vi "Get All Motors.vi"(8 "error in (no error)":errorcluster, 11 "MotionSystem in":refnum<class "MotionSystem.lvclass">) -> (0 "error out":errorcluster, 1 "motors":refnum<class "Motor.lvclass">[](array[class]), 2 "labels":string[](array[string]), 3 "MotionSystem out":refnum<class "MotionSystem.lvclass">)   [LabVIEW 2016, in "MotionSystem.lvlib" / "MotionSystem.lvclass"]
uses:
  <userlib>/Common Components/Hardware/Abstract System/MotionSystem/MotionSystem/MotionSystem.lvclass
  <userlib>/Common Components/Hardware/Motor/Motor/Motor.lvclass
  <userlib>/Common Components/Hardware/Abstract System/MotionSystem/MotionSystem/MotionSystem.lvclass/MotionSystem.ctl
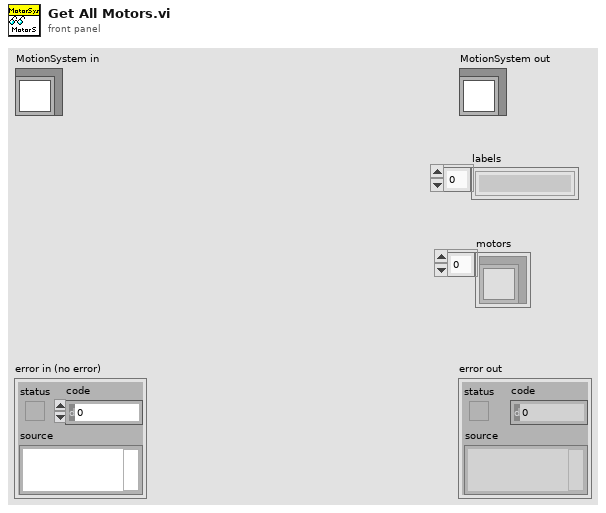
[diagram p1: front panel]
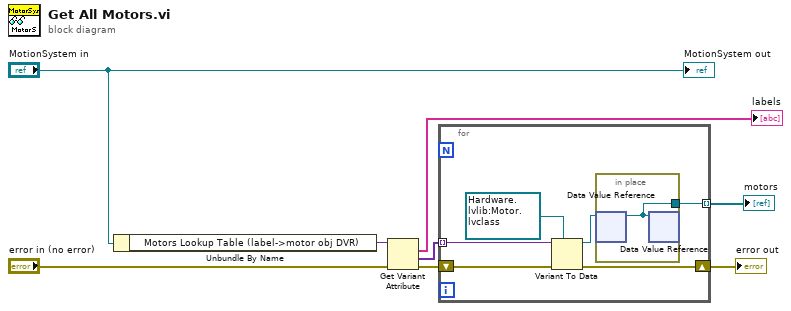
[diagram p0: block diagram]
diagram:
  n1 = Unbundle By Name("MotionSystem in") -> ("Motors Lookup Table (label->motor obj DVR)"=w7:variant)
  n2 = Get Variant Attribute(Variant=w7, error in="error in (no error)") -> (names=→"labels":string[], values=w4:variant[], error out=w3:errorcluster)  [unwired: 2 in, 1 out]
  n3 = for {
    tunnel: w4 -> [w14] mode=indexing
    shift-right: [w12] -> w2
    shift-left: w3 -> [w13]
    tunnel: [w9] -> w1 mode=indexing
    n4 = Variant To Data(error in=w13, type=refnum<data-value> refnum ("data value reference"), Variant=w14) -> (data=w10:refnum<data-value>, error out=w12:errorcluster)
    n5 = in-place {
      in-place-border: [w15] -> w9
      n6 = in-place-dvr #1(w10) -> (w15:refnum<class "Motor.lvclass">)  [unwired: 1 out]
      n7 = in-place-dvr #1(w15) -> ()  [unwired: 2 out]
    }
  }
  "error out" <- w2
  "motors" <- w1
  "MotionSystem out" <- "MotionSystem in"
